vi "PAQmem_FindLatestTimeIndex.vi"(8 "error in (no error)":errorcluster, 11 "PAQ-memory in":refnum<class "PAQ-memory.lvclass">) -> (0 "error out":errorcluster, 1 "Pointer":i32, 2 "Time":timestamp, 3 "PAQ-memory out":refnum<class "PAQ-memory.lvclass">)   [LabVIEW 2020, in "Sgraph_lib_V1.lvlib" / "PAQ-memory.lvclass"]
doc: "Andre Koelewijn, 17 Jan 2021\n\nFind the latest time and index of a PAQ buffer layer"
uses:
  PAQ-memory.lvclass
  PAQ-memory.lvclass/PAQ-memory.ctl
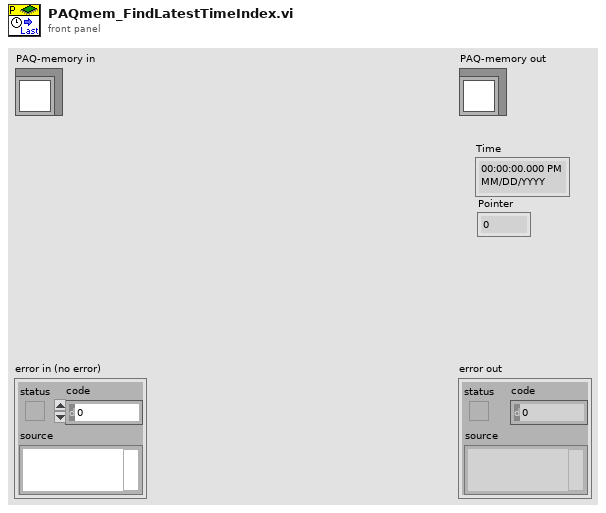
[diagram p1: front panel]
types:
  T1 = typedef "Sgraph_lib_V1.lvlib/FAMM.lvclass/typedef_PAQdata.ctl" = cluster{"TAGs":string[], "Time":refnum<data-value>, "TAGdata":cluster{"source":refnum<data-value>, "status":refnum<data-value>, "data":refnum<data-value>, "max":refnum<data-value>, "min":refnum<data-value>}[]}
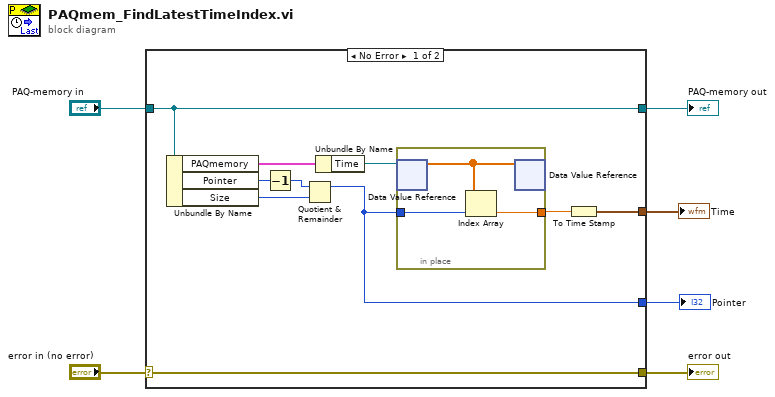
[diagram p0: block diagram]
diagram:
  n1 = case shown="No Error" "error in (no error)" {
    selector: "error in (no error)" -> [w16 w21]
    tunnel: [w16 w21] -> w5
    tunnel: [w13 w20] -> w3
    tunnel: "PAQ-memory in" -> [w13 w20]
    tunnel: [w11 _] -> w2
    tunnel: [w7 _] -> w1
    frame No Error {
      n2 = Unbundle By Name(w13) -> ("PAQmemory"=w15:T1, "Pointer"=w10:i32, "Size"=w9:i32)
      n3 = Decrement(x=w10) -> (x-1=w8:i32)
      n4 = Quotient & Remainder(x=w8, y=w9) -> (x-y*floor(x/y)=w7:i32)  [unwired: 1 out]
      n5 = Unbundle By Name(w15) -> ("Time"=w14:refnum<data-value>)
      n6 = in-place {
        in-place-border: w7 -> [w18]
        in-place-border: [w17] -> w12
        n7 = in-place-dvr #1(w14) -> (w19:dbl[])  [unwired: 1 out]
        n8 = Index Array(array=w19, index=w18) -> (element=w17:dbl)
        n9 = in-place-dvr #1(w19) -> ()  [unwired: 2 out]
      }
      n10 = To Time Stamp(1:w12) -> (0:w11:timestamp)
    }
    frame Error {
    }
  }
  "error out" <- w5
  "PAQ-memory out" <- w3
  "Time" <- w2
  "Pointer" <- w1
